vi "RDMAtoHostDisplay.vi"() -> ()   [LabVIEW 2021]
doc: "Example Description:\nStreams data through host memory from a RIO device then back to the RIO device at the specified rate(s).\n\nVI Configuration:\nThis example uses the PXI-7966R as the FPGA target by default. To use this VI with another FPGA target, use the following steps to configure the host VI to use a VI configured for your FPGA target:\n\n1. On the block diagram, right-click the Open FPGA VI Reference (PXI-7966R) VI and select Configure Open FPGA VI Reference.\n2. Browse for a new target by clicking the Browse Project button in the Open VI section.\n3. Select the VI under the target that matches your device. Click OK to select this VI.\n4. Click OK to exit the dialog box and to apply the new selection to the FPGA VI.\n\nRunning the VI:\n1. Select a RIO Resource that corresponds to the FPGA device configured above.\n2. Configure the Requested host Buffer Depth, Read/Write Size, and Requested (M) controls on the Host VI Front Panel.\n3. Click the run arrow to run the VI.\n4. Observe the Status of the Host Buffer as well as the Input and Output DMA FIFOs\n5. Observe the achieved Streaming Throughput.\n6. Click Stop on the Front Panel to stop the example\n\n\nExecution Steps:\nRefer to the block diagram of the Host VI for each example to view the execution steps for that specific example."
uses:
  utility/decodeToImage/Typedef/PixelFormat.ctl
  <vilib>/rdma/rdma.llb/RDMA Direction.ctl
  <vilib>/rdma/rdma.llb/RDMA Configure Buffers U8.vi
  <vilib>/rdma/rdma.llb/RDMA Acquire Received Buffer U8.vi
  utility/decodeToImage/DecodetoImage.lvlib
panel:
  in  "mS between images":u32=33
  in  "Chunk Size":u32=1048576
  out "Display Error":errorcluster
  out "Frames/s Displayed":dbl
  in  "Image scaling coefficients":dbl[](array[numeric])
  out "Back channel error":errorcluster
  in  "remoteBackChannelPort":u16=50001
  out "General Info and Timing Info":T1={"Block Size w/o Paddings (Bytes)"=12517376, "Frame Count"=1, "Frame Timestamp (ns)"=123, "Lines of Pre-Non-Image Data"=0, "Lines of Image"=2168, "Lines of Post-Non-Image Data"=0, "Bytes per 1st Line"=5772, "Bytes per 2nd Line"=5772, "Image Data Type"=44, "Unused0"=0, "Unused1"=0, "Unused2"=0, "Unused3"=0, "Unused4"=0}
  out "Image":T2(plugin-control)
  out "Total Frames":u32
  in  "Pixel Format":T3
  out "MB/s":dbl format="%#_4f"
  out "Frames/s received":dbl
  in  "Num Host Buffers":u32=10
  out "Image Buffer Size":u32=12513728
  in  "Height":u32=1200
  in  "Width":u32=1920
  in  "localAddress":string="192.168.0.2"
  in  "remotePort":u16=50000
  in  "remoteAddress":string="192.168.0.1"
  out "error out":errorcluster
  in  "Stop":bool
  # "Configuration"
  # "Host"
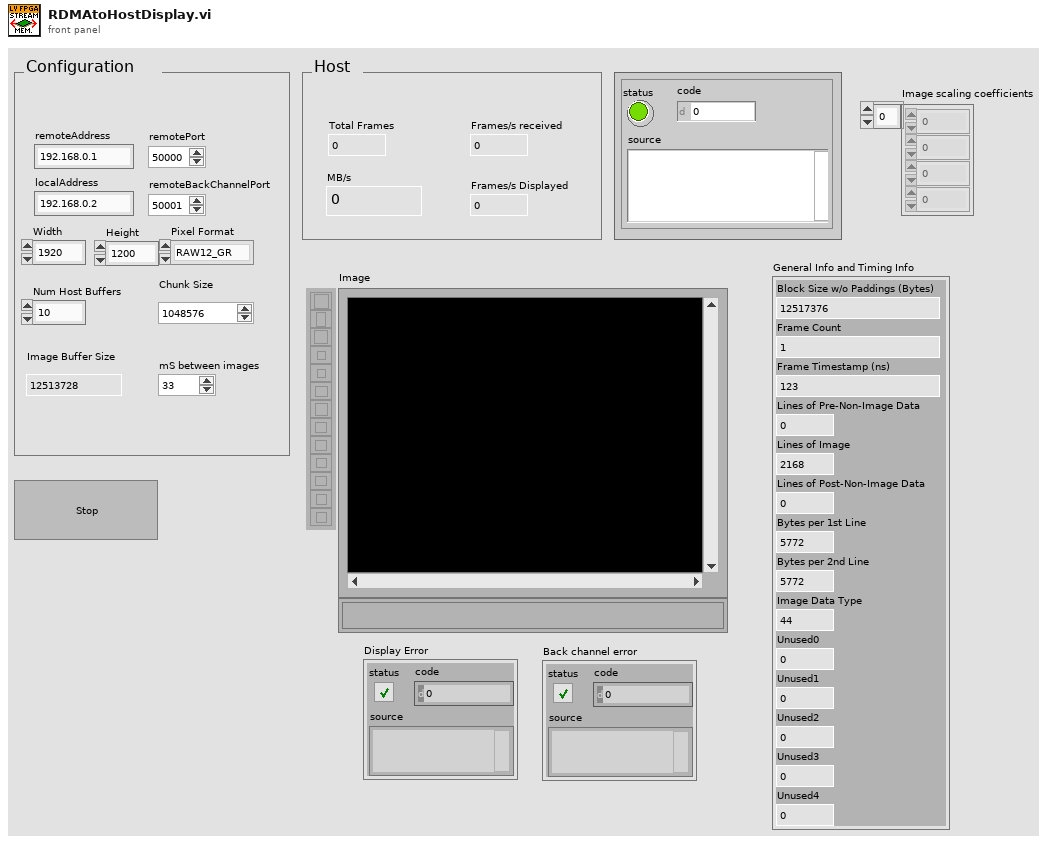
[diagram p1: front panel]
types:
  T1 = cluster{"Block Size w/o Paddings (Bytes)":u32, "Frame Count":u32, "Frame Timestamp (ns)":u64, "Lines of Pre-Non-Image Data":u16, "Lines of Image":u16, "Lines of Post-Non-Image Data":u16, "Bytes per 1st Line":u16, "Bytes per 2nd Line":u16, "Image Data Type":u8, "Unused0":u8, "Unused1":u8, "Unused2":u8, "Unused3":u8, "Unused4":u8}
  T2 = typedef "IMAQ Image.ctl" = refnum<image>
  T3 = typedef "DecodetoImage.lvlib/PixelFormat.ctl" = enum16{"RAW12_GR", "YUV422", "RGB888", "RAW8_GR"}
  T4 = cluster{"Width":u32, "Height":u32, "Properties":cluster{"Pixel Format":T3, "Bits per pixel":i32}}
  T5 = cluster{"Pixel Format":T3, "Bits per pixel":i32}[]
  T6 = typedef "RDMA Direction.ctl" = enum16{"Send", "Receive"}
  T7 = typedef "DecodetoImage.lvlib/Image Transfer Parameters.ctl" = cluster{"Image Queue":refnum<queue>, "Return Queue":refnum<queue>, "Chunk Size":u32, "Frame Fragments":u32, "DVRs":refnum<data-value>[]}
  T8 = enum16{"big-endian, network order", "native, host order", "little-endian"}
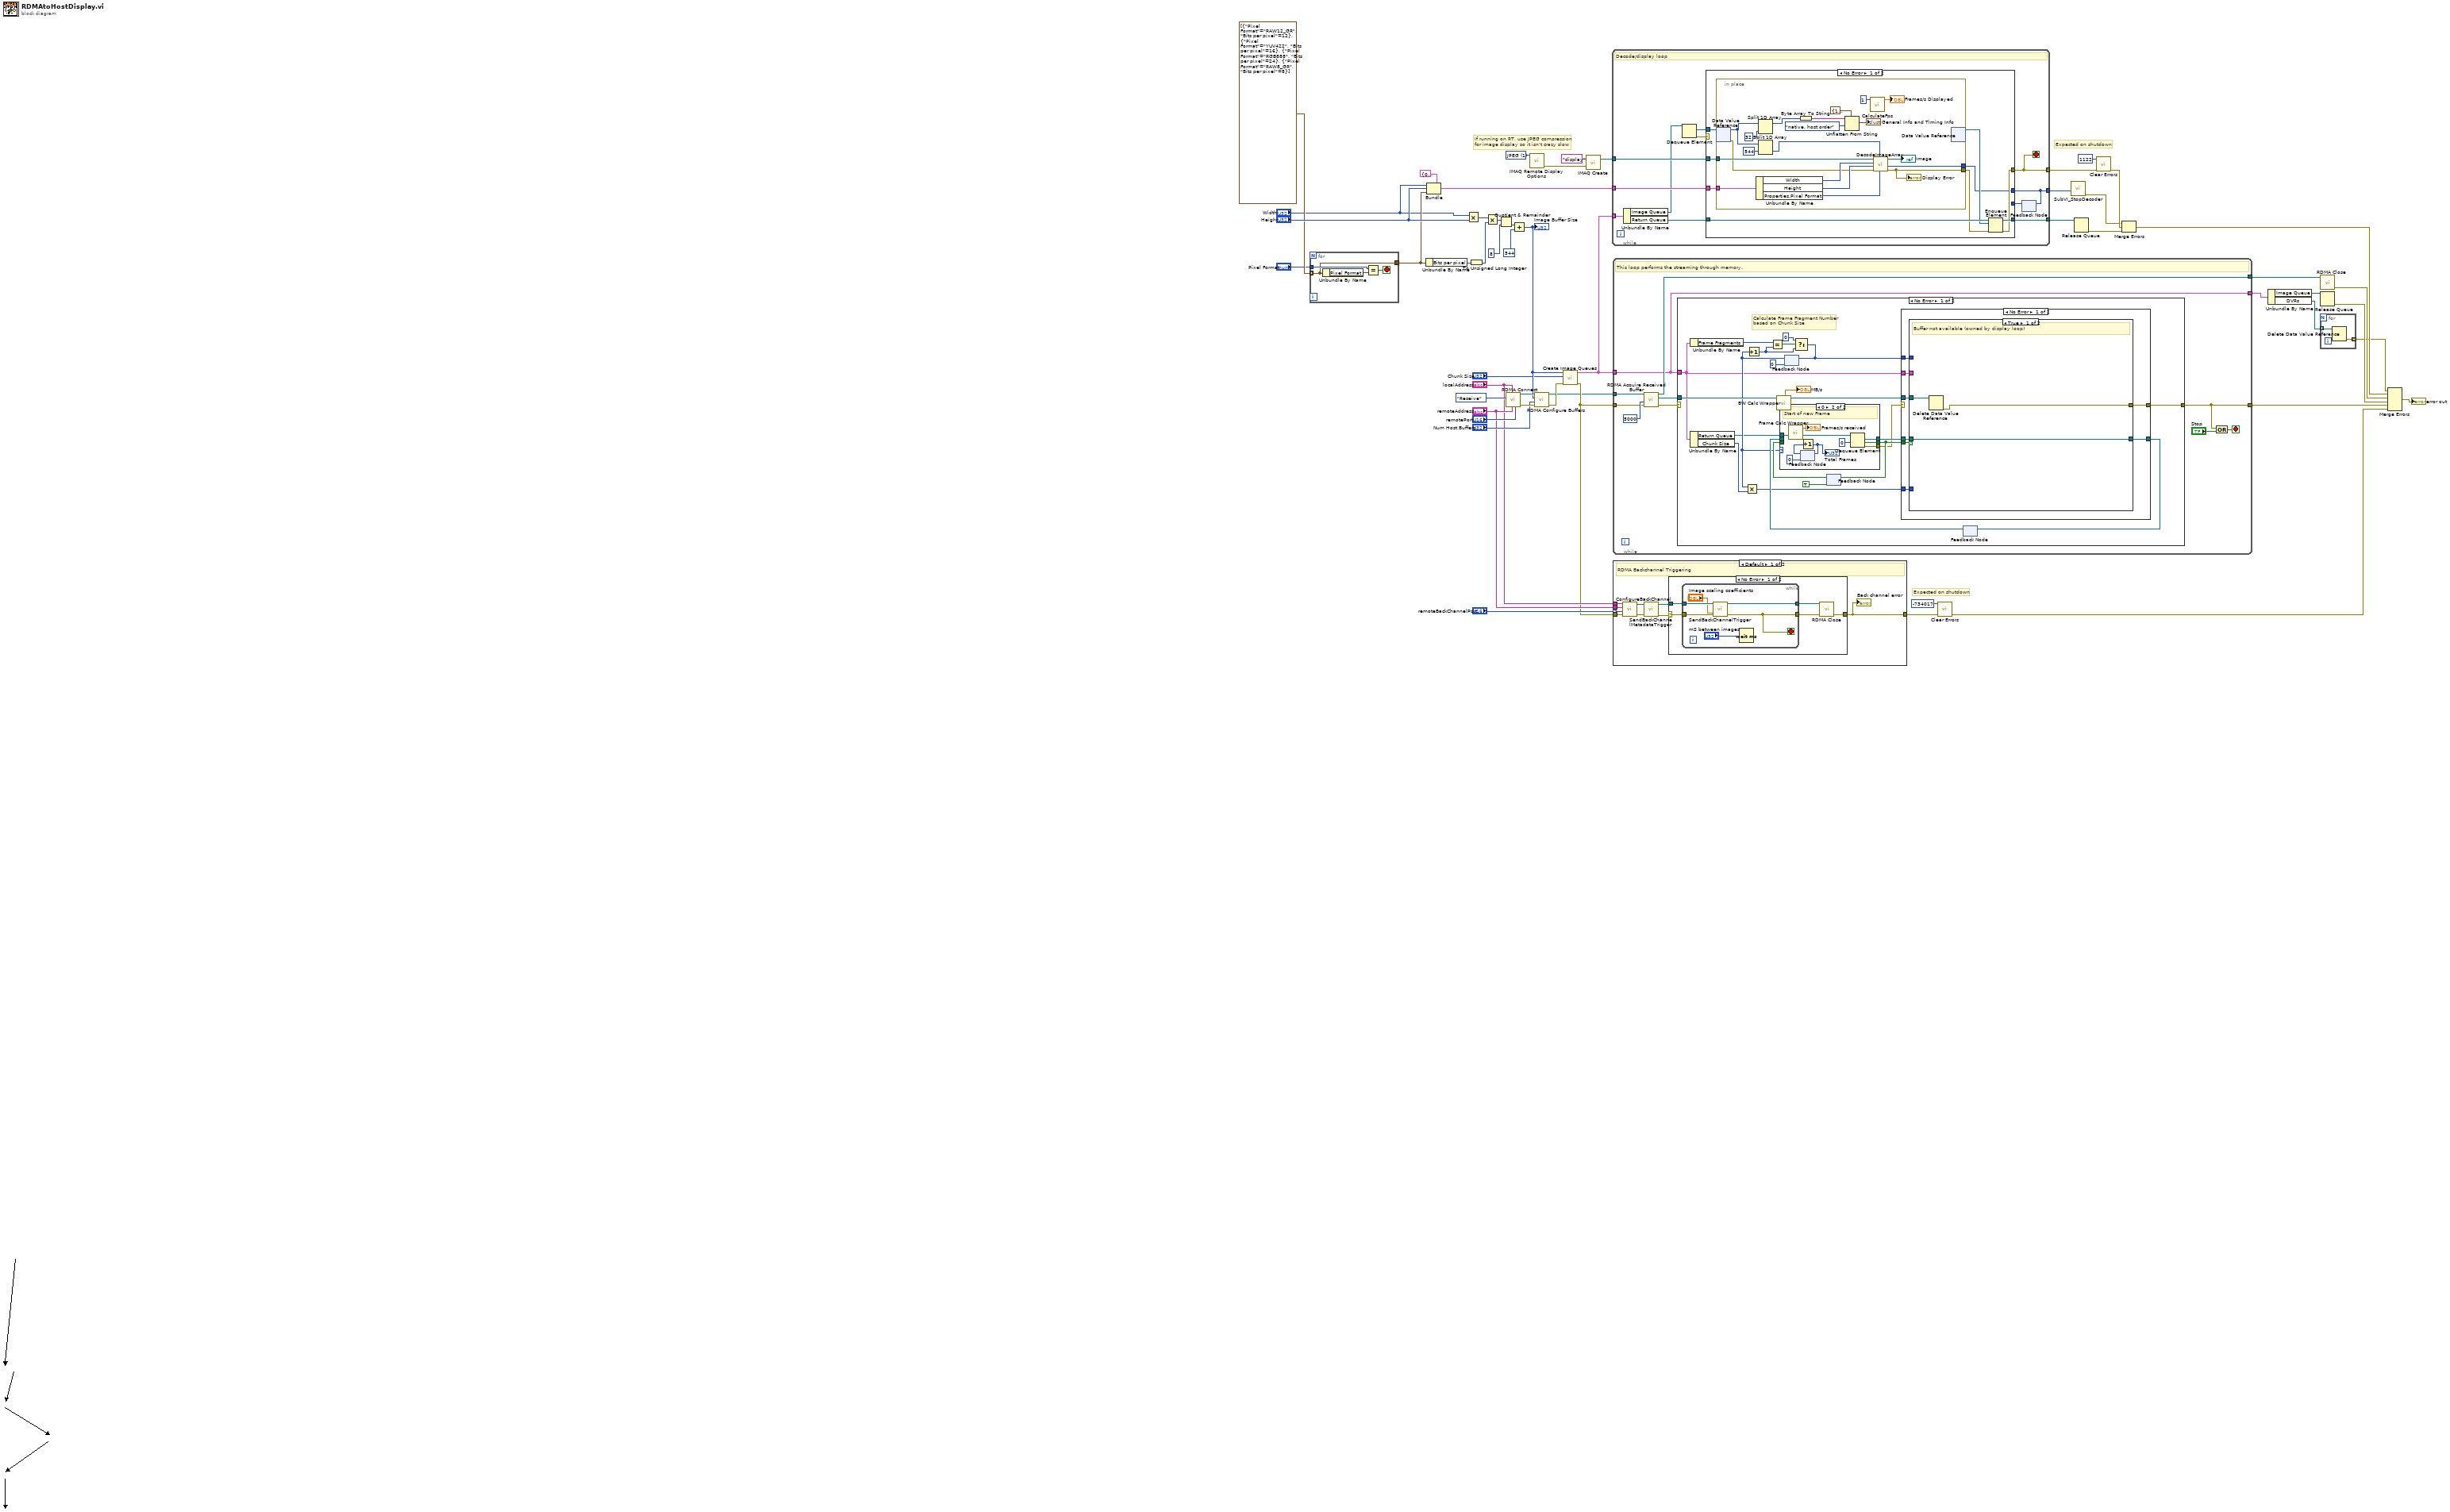
[diagram p0: block diagram]
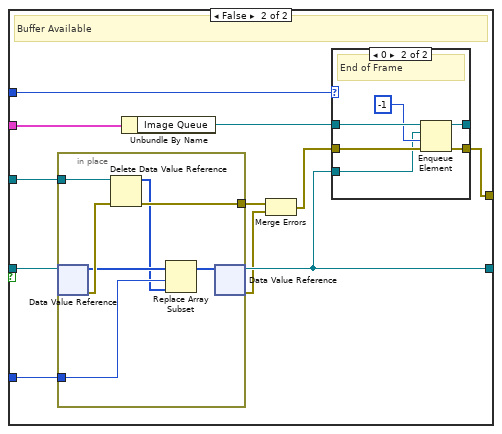
[diagram p2: hidden frame]
diagram:
  w38 = 1 items=["None", "JPEG", "PACKED BINARY"] ("Compression (None)")
  # "Expected on shutdown"
  # "Expected on shutdown"
  # "If running on RT, use JPEG compression\nfor image display so it isn't crazy slow"
  n1 = for {
    tunnel: T5 [{"Pixel Format"=enum."RAW12_GR", "Bits per pixel"=12}, {"Pixel Format"=enum."YUV422", "Bits per pixel"=16}, {"Pixel Format"=enum."RGB888", "Bits per pixel"=24}, {"Pixel Format"=enum."RAW8_GR", "Bits per pixel"=8}] -> [w53] mode=indexing
    tunnel: "Pixel Format" -> [w55]
    tunnel: [w53] -> w40
    stop <- w54 stop-if-true
    n2 = Unbundle By Name(w53) -> ("Pixel Format"=w56:T3)
    n3 = Equal?(x=w55, y=w56) -> (x = y?=w54:bool)
  }
  n4 = Unbundle By Name(w40) -> ("Bits per pixel"=w39:i32)
  n5 = Bundle(cluster=T4 {"Width"=0, "Height"=0, "Properties"={"Pixel Format"=enum."RAW12_GR", "Bits per pixel"=0}}, "Width"="Width", "Height"="Height", "Properties"=w40) -> (w37:T4)
  n6 = Multiply(x="Width", y="Height") -> (x*y=w48:u32)
  n7 = To Unsigned Long Integer(number=w39) -> (unsigned 32bit integer=w21:u32)
  n8 = Multiply(x=w48, y=w21) -> (x*y=w47:u32)
  n9 = Quotient & Remainder(x=w47, y=u32 8) -> (floor(x/y)=w34:u32)  [unwired: 1 out]
  n10 = call <vilib>:"RDMA Connect.vi"("remote port"="remotePort", "remote address"="remoteAddress", "local address"="localAddress", "direction"=RDMA_Direction."Receive") -> ("error out"=w49:errorcluster, "rdma session"=w52:refnum<k21>)  [unwired: 6 in]
  n11 = Add(x=w34, y=u32 544) -> (x+y=w19:u32)
  "Image Buffer Size" <- w19
  n12 = call "IMAQ Remote Display Options"("Compression (None)"=w38) -> ("error out"=w28:errorcluster)  [unwired: 8 in, 2 out]
  n13 = call-poly <vilib>:"RDMA Configure Buffers.vi"("error in"=w49, "max concurrent transactions"="Num Host Buffers", "max transaction size"=w19, "rdma session in"=w52) -> ("error out"=w29:errorcluster, "rdma session out"=w14:refnum<k21>)  [unwired: 6 in]
  n14 = call "Create Image Queues.vi"("error in (no error)"=w29, "Chunk Size"="Chunk Size", "Image Size"=w19) -> ("error out"=w20:errorcluster, "Image Transfer Parameters"=w17:T7)  [unwired: 7 in]
  n15 = call "IMAQ Create"("Image Name"="display", "error in (no error)"=w28) -> ("New Image"=w35:T2)  [unwired: 3 in, 1 out]
  n16 = while {
    tunnel: w17 -> [w61]
    tunnel: w37 -> [w67]
    tunnel: w35 -> [w66]
    tunnel: [w65] -> w23
    tunnel: [w63] -> w4
    tunnel: [w58] -> w5
    stop <- w65 stop-if-true
    # "Decode/display loop"
    n17 = Unbundle By Name(w61) -> ("Image Queue"=w59:refnum<queue>, "Return Queue"=w60:refnum<queue>)
    n18 = Dequeue Element(queue=w59) -> (element=w64:refnum<data-value>, error out=w62:errorcluster)  [unwired: 2 in, 2 out]
    n19 = feedback #1() -> (w57:u64)  [unwired: 1 in]
    n20 = case shown="No Error" w62 {
      selector: w62 -> [_ w99]
      tunnel: w67 -> [w76 _]
      tunnel: w66 -> [w75 _]
      tunnel: [w71 w99] -> w65
      tunnel: w64 -> [w74 _]
      tunnel: w60 -> [w73 w98]
      tunnel: [w72 w98] -> w63
      tunnel: [w68 w97] -> w58
      tunnel: w57 -> [_ w97]
      frame No Error {
        n21 = in-place {
          in-place-border: w76 -> [w96]
          in-place-border: w75 -> [w95]
          in-place-border: [w85] -> w69
          in-place-border: [w81] -> w68
          n22 = in-place-dvr #2(w74) -> (w78:u8[], w84:errorcluster)
          n23 = Unbundle By Name(w96) -> ("Width"=w88:u32, "Height"=w87:u32, "Properties.Pixel Format"=w94:T3)
          n24 = Split 1D Array(array=w78, index=32) -> (first subarray=w86:u8[])  [unwired: 1 out]
          n25 = Split 1D Array(array=w78, index=544) -> (second subarray=w77:u8[])  [unwired: 1 out]
          n26 = Byte Array To String(unsigned byte array=w86) -> (string=w91:string)
          n27 = Unflatten From String(type=T1 {"Block Size w/o Paddings (Bytes)"=12517376, "Frame Count"=1, "Frame Timestamp (ns)"=123, "Lines of Pre-Non-Image Data"=0, "Lines of Image"=2168, "Lines of Post-Non-Image Data"=0, "Bytes per 1st Line"=5772, "Bytes per 2nd Line"=5772, "Image Data Type"=44, "Unused0"=0, "Unused1"=0, "Unused2"=0, "Unused3"=0, "Unused4"=0} ("General Info and Timing Info 2"), binary string=w91, byte order (0:big-endian, network order)=T8."native, host order") -> (value=→"General Info and Timing Info":T1)  [unwired: 2 in, 2 out]
          n28 = call "CalculateFps.vi"("New Frames Transferred"=u64 1) -> ("Frames/s"=→"Frames/s Displayed":dbl)  [unwired: 10 in]
          n29 = call "DecodeImageArray.vi"("Pixel Format"=w94, "Source Image In"=w77, "error in (no error)"=w84, "Height"=w87, "Width"=w88, "image  in"=w95) -> ("error out"=w85:errorcluster, "decoder out"=w81:u64, "image out"=→"Image":T2)  [unwired: 2 in, 1 out]
          "Display Error" <- w85
          n30 = in-place-dvr #2() -> (w70:refnum<data-value>)  [unwired: 1 in, 1 out]
        }
        n31 = Enqueue Element(queue=w73, element=w70, error in (no error)=w69) -> (queue out=w72:refnum<queue>, error out=w71:errorcluster)  [unwired: 1 in, 1 out]
      }
      frame Error {
      }
    }
    n32 = feedback-in #1(w58) -> ()
  }
  n33 = while {
    tunnel: w20 -> [w102]
    tunnel: w14 -> [w107]
    tunnel: [w106] -> w8
    tunnel: w17 -> [w100]
    tunnel: [w100] -> w12
    tunnel: [w101] -> w13
    stop <- w108 stop-if-true
    # "This loop performs the streaming through memory."
    n34 = call-poly <vilib>:"RDMA Acquire Received Buffer.vi"("error in"=w102, "timeout (ms)"=5000, "rdma session in"=w107) -> ("error out"=w104:errorcluster, "edvr"=w103:refnum<data-value>, "rdma session out"=w101:refnum<k21>)  [unwired: 6 in]
    n35 = case shown="No Error" w104 {
      selector: w104 -> [_ w182]
      tunnel: w103 -> [w131 _]
      tunnel: [w114 w182] -> w106
      tunnel: w100 -> [w110 _]
      frame No Error {
        # "Calculate Frame Fragment Number based on Chunk Size"
        # "Buffer up to single frame for decode/display, otherwise return references immediately."
        n36 = Unbundle By Name(w110) -> ("Frame Fragments"=w113:u32)
        n37 = Unbundle By Name(w110) -> ("Return Queue"=w112:refnum<queue>, "Chunk Size"=w111:u32)
        n38 = call "BW Calc Wrapper.vi"("Data Value Reference in"=w131) -> ("MB/s"=→"MB/s":dbl, "Data Value Reference out"=w130:refnum<data-value>)  [unwired: 2 in]
        n39 = feedback #3(u32 0 ("timeout in ms (-1)")) -> (w116:u32)
        n40 = Multiply(x=w116, y=w111) -> (x*y=w117:u32)
        n41 = Increment(x=w116) -> (x+1=w126:u32)
        n42 = Equal?(x=w113, y=w126) -> (x = y?=w127:bool)
        n43 = Select(t=u32 0, s=w127, f=w126) -> (s? t:f=w119:u32)
        n44 = feedback-in #3(w119) -> ()
        n45 = feedback #4(TRUE ("timed out?")) -> (w122:bool)
        n46 = feedback #5() -> (w120:refnum<data-value>)  [unwired: 1 in]
        n47 = case shown="0" w116 {
          tunnel: w112 -> [_ w181]
          tunnel: [w172 w180] -> w118
          tunnel: [w171 w179] -> w128
          tunnel: w122 -> [w172 _]
          tunnel: w120 -> [w171 _]
          tunnel: [_ w173] -> w115
          frame 1, Default {
          }
          frame 0 {
            # "Start of new Frame"
            n48 = call "Frame Calc Wrapper.vi"() -> ("Frames/s received"=→"Frames/s received":dbl)  [unwired: 5 in]
            n49 = feedback #6(u32 0 ("timeout in ms (-1)")) -> (w175:u32)
            n50 = Increment(x=w175) -> (x+1=w176:u32)
            "Total Frames" <- w176
            n51 = feedback-in #6(w176) -> ()
            n52 = Dequeue Element(queue=w181, timeout in ms (-1)=0) -> (element=w179:refnum<data-value>, timed out?=w180:bool, error out=w173:errorcluster)  [unwired: 1 in, 1 out]
          }
        }
        n53 = feedback-in #4(w118) -> ()
        n54 = case shown="No Error" w115 {
          selector: w115 -> [_ w170]
          tunnel: w130 -> [w139 _]
          tunnel: w110 -> [w138 _]
          tunnel: w128 -> [w137 w169]
          tunnel: [w136 w169] -> w121
          tunnel: w119 -> [w135 _]
          tunnel: w118 -> [w134 _]
          tunnel: w117 -> [w133 _]
          tunnel: [w132 w170] -> w114
          frame No Error {
            n55 = case shown="True" w134 {
              tunnel: w139 -> [w142 w152]
              tunnel: w138 -> [_ w144]
              tunnel: w137 -> [w141 w153]
              tunnel: [w141 w150] -> w136
              tunnel: w135 -> [_ w149]
              tunnel: w133 -> [_ w148]
              tunnel: [w140 w145] -> w132
              frame True {
                # "Buffer not available (owned by display loop)"
                n56 = Delete Data Value Reference(data value reference=w142) -> (error out=w140:errorcluster)  [unwired: 1 in, 1 out]
              }
              frame False {
                # "Buffer Available"
                n57 = in-place {
                  in-place-border: w152 -> [w168]
                  in-place-border: [w167] -> w147
                  in-place-border: w148 -> [w164]
                  n58 = in-place-dvr #7(w153) -> (w165:u8[], w166:errorcluster)
                  n59 = Delete Data Value Reference(data value reference=w168, error in=w166) -> (data value=w163:u8[], error out=w167:errorcluster)
                  n60 = Replace Array Subset(array=w165, new element=w163, index=w164) -> (w162:u8[])
                  n61 = in-place-dvr #7(w162) -> (w150:refnum<data-value>, w146:errorcluster)
                }
                n62 = Unbundle By Name(w144) -> ("Image Queue"=w143:refnum<queue>)
                n63 = Merge Errors(w147, w146) -> (w151:errorcluster)
                n64 = case shown="0" w149 {
                  tunnel: w143 -> [w155 w161]
                  tunnel: [w155 w159] -> _
                  tunnel: w151 -> [w154 w158]
                  tunnel: w150 -> [_ w157]
                  tunnel: [w154 w156] -> w145
                  frame 1, Default {
                  }
                  frame 0 {
                    # "End of Frame"
                    n65 = Enqueue Element(queue=w161, element=w157, timeout in ms (-1)=-1, error in (no error)=w158) -> (queue out=w159:refnum<queue>, error out=w156:errorcluster)  [unwired: 1 out]
                  }
                }
              }
            }
          }
          frame Error {
          }
        }
        n66 = feedback-in #5(w121) -> ()
      }
      frame Error {
      }
    }
    n67 = Compound Arithmetic op=OR(w106, "Stop") -> (w108:bool)
  }
  n68 = case shown="Default" "remoteBackChannelPort" {
    selector: "remoteBackChannelPort" -> [w191 _]
    tunnel: w20 -> [w190 w204]
    tunnel: "remoteAddress" -> [w189 _]
    tunnel: "localAddress" -> [w188 _]
    tunnel: [w187 w204] -> w24
    frame Default {
      # "RDMA Backchannel Triggering"
      n69 = call "ConfigureBackChannel.vi"("error in"=w190, "backchannel remote port"=w191, "remote address"=w189, "local address"=w188) -> ("error out"=w186:errorcluster, "rdma session out"=w184:refnum<k21>)  [unwired: 6 in]
      n70 = call "SendBackChannelMetadataTrigger.vi"("error in"=w186, "rdma session in"=w184) -> ("error out"=w183:errorcluster, "rdma session out"=w185:refnum<k21>)  [unwired: 8 in]
      n71 = case shown="No Error" w183 {
        selector: w183 -> [w195 w203]
        tunnel: w185 -> [w196 _]
        tunnel: [w192 w203] -> w187
        frame No Error {
          n72 = while {
            tunnel: w196 -> [w201]
            tunnel: w195 -> [w200]
            tunnel: [w199] -> w194
            tunnel: [w198] -> w193
            stop <- w198 stop-if-true
            n73 = call "SendBackChannelTrigger.vi"("Image scaling coefficients"="Image scaling coefficients", "error in"=w200, "rdma session in"=w201) -> ("error out"=w198:errorcluster, "rdma session out"=w199:refnum<k21>)  [unwired: 7 in]
            n74 = Wait (ms)(milliseconds to wait="mS between images") -> ()  [unwired: 1 out]
          }
          n75 = call <vilib>:"RDMA Close.vi"("error in"=w193, "rdma session"=w194) -> ("error out"=w192:errorcluster)  [unwired: 9 in]
        }
        frame Error {
        }
      }
      "Back channel error" <- w187
    }
    frame 0 {
    }
  }
  n76 = call <vilib>:"Clear Errors.vi"("error in (no error)"=w24, "specific error code to clear (0: all)"=-734017) -> ("error out"=w7:errorcluster)  [unwired: 4 in, 1 out]
  n77 = call "SubVI_StopDecoder.vi"("decoder in"=w5) -> ("error"=w6:errorcluster)  [unwired: 10 in]
  n78 = Release Queue(queue=w4) -> (error out=w3:errorcluster)  [unwired: 2 in, 2 out]
  n79 = call <vilib>:"Clear Errors.vi"("error in (no error)"=w23, "specific error code to clear (0: all)"=1122) -> ("error out"=w15:errorcluster)  [unwired: 4 in, 1 out]
  n80 = Merge Errors(w6, w15, w3) -> (w10:errorcluster)
  n81 = Unbundle By Name(w12) -> ("Image Queue"=w11:refnum<queue>, "DVRs"=w2:refnum<data-value>[])
  n82 = for {
    tunnel: w2 -> [w206] mode=indexing
    tunnel: [w205] -> w1 mode=indexing
    n83 = Delete Data Value Reference(data value reference=w206) -> (error out=w205:errorcluster)  [unwired: 1 in, 1 out]
  }
  n84 = call <vilib>:"RDMA Close.vi"("rdma session"=w13) -> ("error out"=w9:errorcluster)  [unwired: 10 in]
  n85 = Release Queue(queue=w11) -> (error out=w16:errorcluster)  [unwired: 2 in, 2 out]
  n86 = Merge Errors(w1, w10, w9, w16, w8, w7) -> (→"error out":errorcluster)
